vi "Bin Winch Interface.vi"(11 "Winch Command":T1(ring)=enum."Hold") -> ()   [LabVIEW 2014]
panel:
  in  "Desired Height":dbl
  out "Drive Output":dbl=-0.08058785684999847 format="%#_4f"
  in  "Kp":dbl=1.0
  in  "Reset Encoder?":bool
  out "Stopped":bool=TRUE
  out "Rate":dbl format="%#_4f"
  out "Direction":bool
  out "Distance":dbl=30.619144136850004 format="%#_5f"
  in  "Max Winch Drive Torque":dbl=1.0 format="%#_13g"
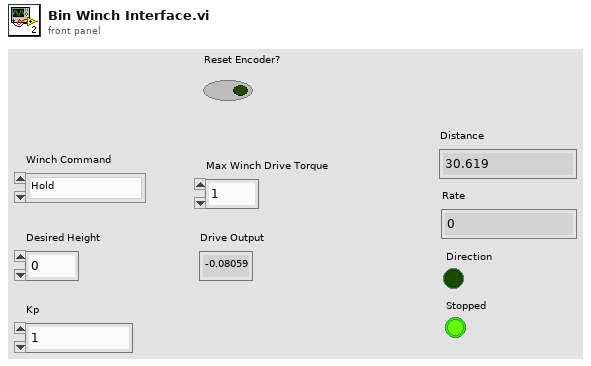
[diagram p1: front panel]
types:
  T1 = enum16{"Position Bottom", "Off", "Hold", "Jog Down", "Jog Up", "Position Top", ""}
  T2 = typedef "WPI_DigitalInputDevRef.ctl" = cluster{"DevStatus":errorcluster, "DIO Channel":T3, "Controller":T4}
  T3 = typedef "FPGA_DIOChannel.ctl" = enum8{"DIO 0", "DIO 1", "DIO 2", "DIO 3", "DIO 4", "DIO 5", "DIO 6", "DIO 7", "DIO 8", "DIO 9", "DIO MXP 0", "DIO MXP 1", "DIO MXP 2", "DIO MXP 3", "DIO MXP 4", "DIO MXP 5", "DIO MXP 6", "DIO MXP 7", "DIO MXP 8", "DIO MXP 9", "DIO MXP 10", "DIO MXP 11", "DIO MXP 12", "DIO MXP 13", "DIO MXP 14", "DIO MXP 15", "Invalid"}
  T4 = typedef "FPGA_TypedefDigitalModule.ctl" = enum16{"Controller 1"}
  T5 = typedef "WPI_EncoderDevRef.ctl" = cluster{"DevStatus":errorcluster, "EncoderIndex":T6, "CounterIndex":T7, "DistancePerCount":dbl, "Decoding Type":T8}
  T6 = typedef "FPGA_EncoderIdx.ctl" = enum8{"Enc 0", "Enc 1", "Enc 2", "Enc 3", "Enc 4", "Enc 5", "Enc 6", "Enc 7", "Invalid"}
  T7 = typedef "FPGA_CounterCtrSystemIndex.ctl" = enum8{"Ctr 0", "Ctr 1", "Ctr 2", "Ctr 3", "Ctr 4", "Ctr 5", "Ctr 6", "Ctr 7", "Invalid"}
  T8 = typedef "WPI_EncoderType.ctl" = enum16{"1x", "2x", "4x"}
  T9 = typedef "WPI_MotorControlDeviceRef.ctl" = cluster{"DeviceStatus":errorcluster, "Type":T10, "PWM":cluster{"Controller":T4, "PWM Channel":T11, "DeadBand":T12}, "CAN":cluster{"Device Number":u8, "Control Mode":T13, "Semaphore":T14, "Max Vout":dbl, "TalonSRX Control Mode":T15}, "Invert":bool, "TransformRef":T16, "InvTransformRef":T16}
  T10 = typedef "WPI_MotorControlType.ctl" = enum16{"PWM", "CAN", "CANTalonSRX"}
  T11 = typedef "FPGA_DIOPWMChannel.ctl" = enum8{"PWM 0", "PWM 1", "PWM 2", "PWM 3", "PWM 4", "PWM 5", "PWM 6", "PWM 7", "PWM 8", "PWM 9", "PWM MXP 0", "PWM MXP 1", "PWM MXP 2", "PWM MXP 3", "PWM MXP 4", "PWM MXP 5", "PWM MXP 6", "PWM MXP 7", "PWM MXP 8", "PWM MXP 9", "Invalid"}
  T12 = typedef "WPI_PWMDeadband.ctl" = cluster{"Name":string, "maxPositivePwm":i32, "minPositivePwm":i32, "centerPwm":i32, "maxNegativePwm":i32, "minNegativePwm":i32, "angularRange":u16}
  T13 = typedef "WPI_CANJaguar_ControlMode.ctl" = enum8{"Percent VBus", "Current", "Speed", "Position", "Voltage"}
  T14 = typedef "Semaphore RefNum" = refnum<k1>
  T15 = typedef "WPI_CANTalonSRX_APIControlMode.ctl" = enum8{"Percent VBus", "Speed", "Position", "Slave", "Unchanged / Invalid"}
  T16 = typedef "WPI_PWMTransform_ConPane.ctl" = refnum<vi>
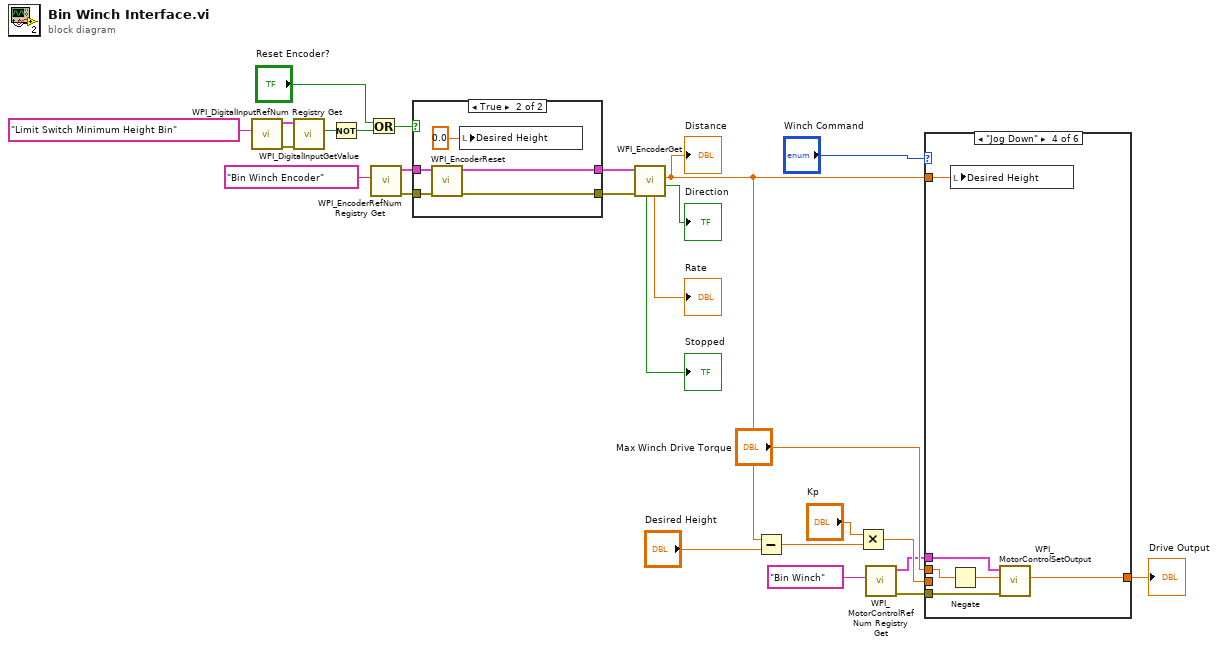
[diagram p0: block diagram]
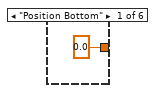
[diagram p3: hidden frame]
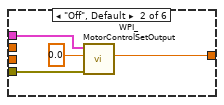
[diagram p4: hidden frame]
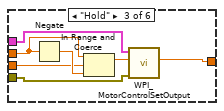
[diagram p5: hidden frame]
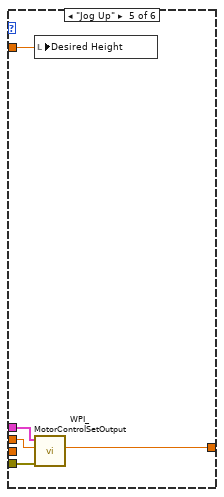
[diagram p6: hidden frame]
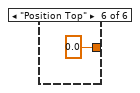
[diagram p7: hidden frame]
diagram:
  n1 = call <vilib>:"WPI_DigitalInputRefNum Registry Get.vi"("refnum name"="Limit Switch Minimum Height Bin") -> ("error out"=w7:errorcluster, "DigitalInputDevRef"=w8:T2)  [unwired: 9 in]
  n2 = call <vilib>:"WPI_DigitalInputGetValue.vi"("error in (no error)"=w7, "DigitalInputDevRef"=w8) -> ("Value"=w3:bool)  [unwired: 7 in, 2 out]
  n3 = Not(x=w3) -> (.not. x?=w2:bool)
  n4 = Or(x="Reset Encoder?", y=w2) -> (x .or. y?=w4:bool)
  n5 = call <vilib>:"WPI_EncoderRefNum Registry Get.vi"("refnum name"="Bin Winch Encoder") -> ("error out"=w19:errorcluster, "EncoderDevRef"=w20:T5)  [unwired: 9 in]
  n6 = case shown="True" w4 {
    tunnel: w20 -> [w28 w33]
    tunnel: w19 -> [w27 w32]
    tunnel: [w27 w31] -> w18
    tunnel: [w28 w30] -> w17
    frame False {
    }
    frame True {
      n7 = call <vilib>:"WPI_EncoderReset.vi"("error in (no error)"=w32, "EncoderDevRef"=w33) -> ("error out"=w31:errorcluster, "EncoderDevRef"=w30:T5)  [unwired: 8 in]
      n8 = local write "Desired Height"(0.0 ("Desired Height")) -> ()
    }
  }
  n9 = call <vilib>:"WPI_EncoderGet.vi"("error in (no error)"=w18, "EncoderDevRef"=w17) -> ("Direction"=→"Direction":bool, "Distance"=w9:dbl, "Rate"=→"Rate":dbl, "Stopped"=→"Stopped":bool)  [unwired: 4 in, 2 out]
  "Distance" <- w9
  n10 = Subtract(x=w9, y="Desired Height") -> (x-y=w14:dbl)
  n11 = Multiply(x="Kp", y=w14) -> (x*y=w12:dbl)
  n12 = call <vilib>:"WPI_MotorControlRefNum Registry Get.vi"("refnum name"="Bin Winch") -> ("error out"=w10:errorcluster, "MotorControlDevRef"=w11:T9)  [unwired: 9 in]
  n13 = case shown="\"Jog Down\"" "Winch Command" {
    tunnel: "Max Winch Drive Torque" -> [_ _ w43 w50 w56 _]
    tunnel: w11 -> [_ w37 w45 w49 w55 _]
    tunnel: w10 -> [_ w36 w44 w48 w54 _]
    tunnel: w12 -> [_ _ w41 _ _ _]
    tunnel: w9 -> [_ _ _ w47 w53 _]
    tunnel: [0.0 ("Motor Output") w35 w39 w46 w52 0.0 ("Motor Output")] -> w1
    frame "Position Bottom" {
    }
    frame "Off", Default {
      n14 = call <vilib>:"WPI_MotorControlSetOutput.vi"("error in (no error)"=w36, "Output"=0.0 ("Motor Output"), "MotorControlDevRef"=w37) -> ("Motor Output"=w35:dbl)  [unwired: 6 in, 2 out]
    }
    frame "Hold" {
      n15 = Negate(x=w43) -> (-x=w42:dbl)
      n16 = In Range and Coerce(upper limit=w43, x=w41, lower limit=w42) -> (coerced(x)=w40:dbl)  [unwired: 1 out]
      n17 = call <vilib>:"WPI_MotorControlSetOutput.vi"("error in (no error)"=w44, "Output"=w40, "MotorControlDevRef"=w45) -> ("Motor Output"=w39:dbl)  [unwired: 6 in, 2 out]
    }
    frame "Jog Down" {
      n18 = Negate(x=w50) -> (-x=w51:dbl)
      n19 = local write "Desired Height"(w47) -> ()
      n20 = call <vilib>:"WPI_MotorControlSetOutput.vi"("error in (no error)"=w48, "Output"=w51, "MotorControlDevRef"=w49) -> ("Motor Output"=w46:dbl)  [unwired: 6 in, 2 out]
    }
    frame "Jog Up" {
      n21 = local write "Desired Height"(w53) -> ()
      n22 = call <vilib>:"WPI_MotorControlSetOutput.vi"("error in (no error)"=w54, "Output"=w56, "MotorControlDevRef"=w55) -> ("Motor Output"=w52:dbl)  [unwired: 6 in, 2 out]
    }
    frame "Position Top" {
    }
  }
  "Drive Output" <- w1
